vi "Set Positions.vi"(8 "error in":errorcluster, 9 "Type of Neuron":T1=enum."GC", 11 "Grid in":refnum<class "Grid.lvclass">) -> (0 "error out":errorcluster, 3 "Grid out":refnum<class "Grid.lvclass">)   [LabVIEW 2016, in "Grid.lvclass"]
doc: "This Vi perform the random allocation of #(No Nodes) inside the 3D grid of dimensions (Size(um)), accodring to the boundaries given by the Layer. Granular layer is confined to 80% in the Z dimension. Purkinje/Molecular layer is confined to 20% of the Z dimension."
uses:
  Grid.lvclass
  Controls/Type of Neuron.ctl
  Grid.lvclass/Grid.ctl
  Controls/SM Allocate Neurons.ctl
  Neuron/Neuron.lvclass/Neuron.ctl
  Neuron/Neuron.lvclass
panel:
  out "Iteration No":i32
  out "Neurons Allocated":i32
  out "Avai Ids":i32
  out "Ids Neighboor":i32[](array[numeric])
  out "Riffled {Ids}":i32[](array[numeric])
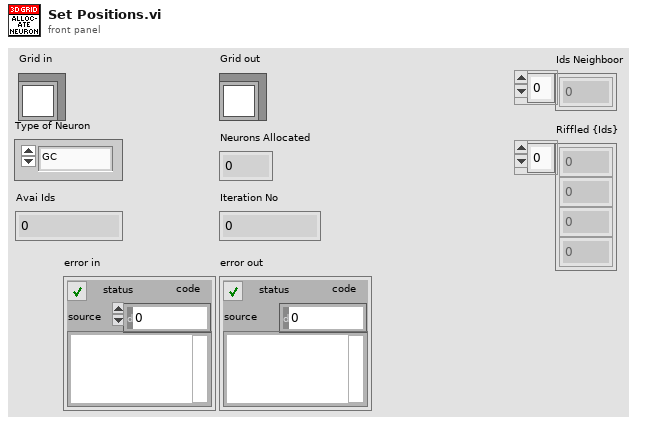
[diagram p1: front panel]
types:
  T1 = typedef "Type of Neuron.ctl" = enum16{"MF", "BA", "GO", "GC", "PC", "LU", "Glia (Dummy)"}
  T2 = typedef "SM Allocate Neurons.ctl" = enum16{"Initialize", "Generate ID", "Check Perifery", "Ocuppy it", "Stop"}
  T3 = typedef "Neuron Info.ctl" = cluster{"N":i32, "Radius":dbl, "Type":T1, "Color":u32}[]
  T4 = cluster{"N":i32, "Radius":dbl, "Type":T1, "Color":u32}
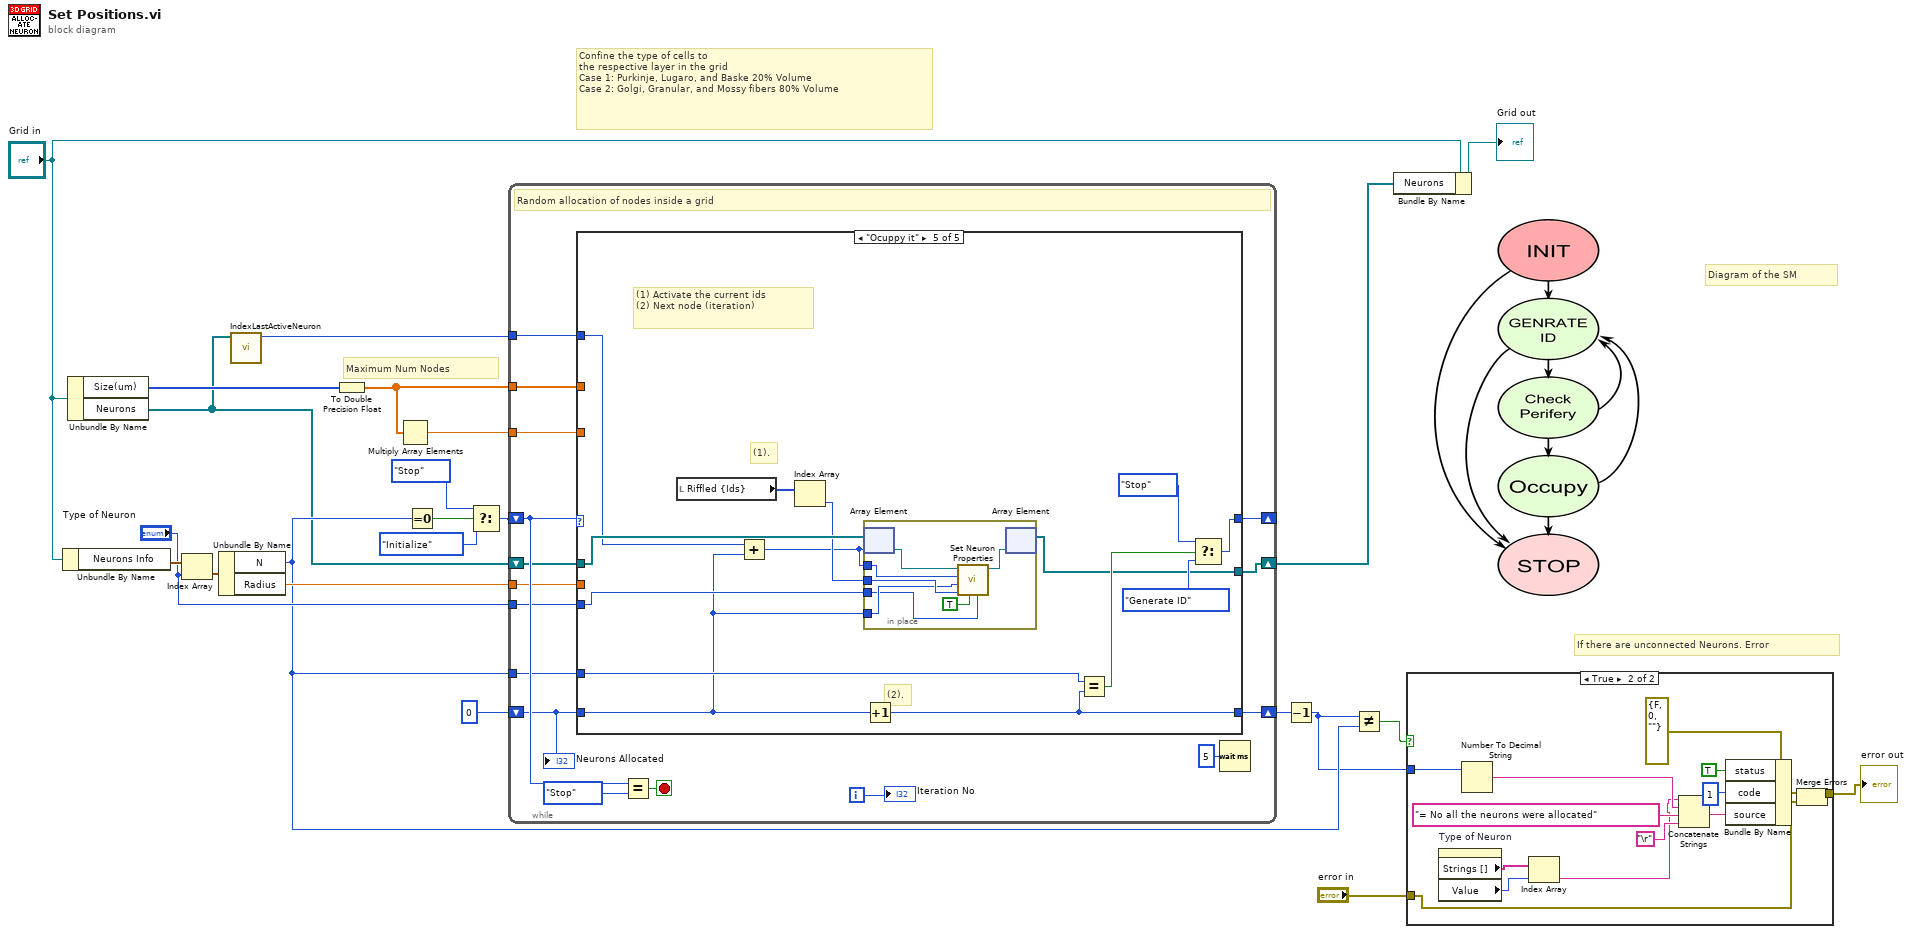
[diagram p0: block diagram]
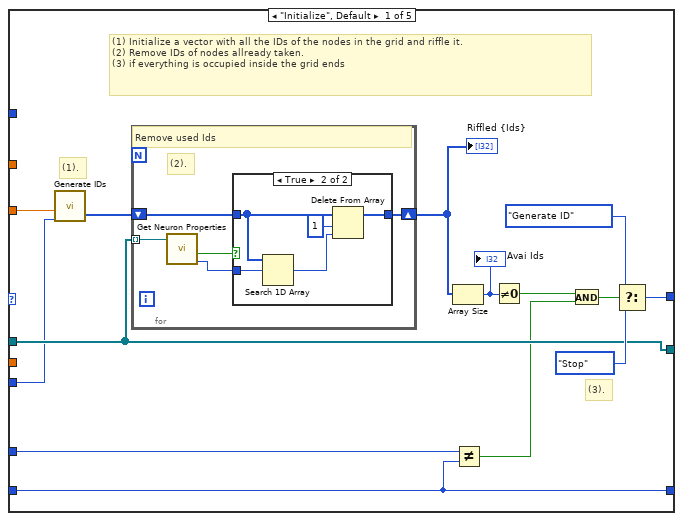
[diagram p3: hidden frame]
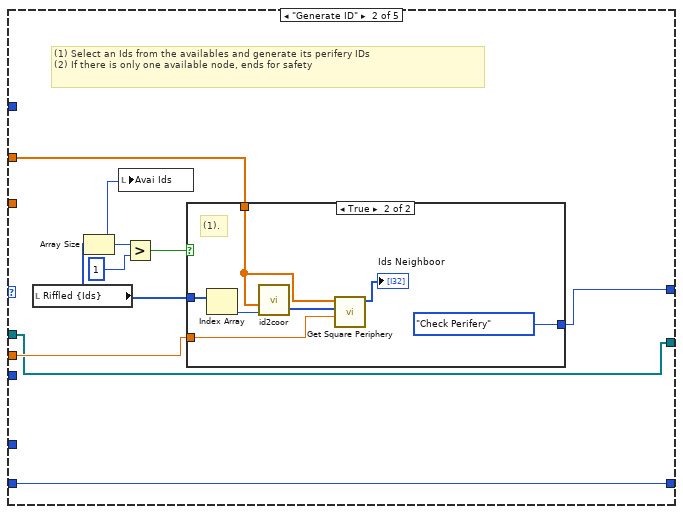
[diagram p5: hidden frame]
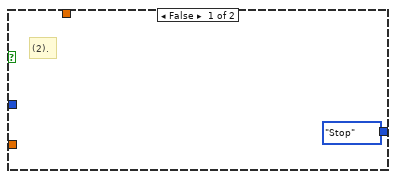
[diagram p6: hidden frame]
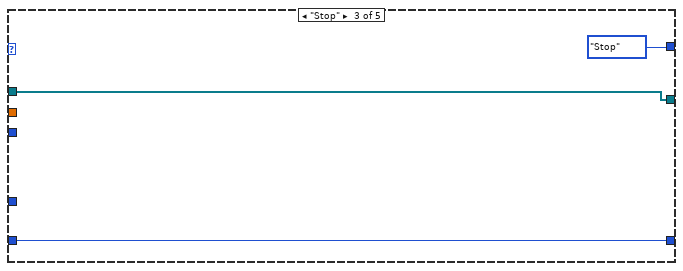
[diagram p7: hidden frame]
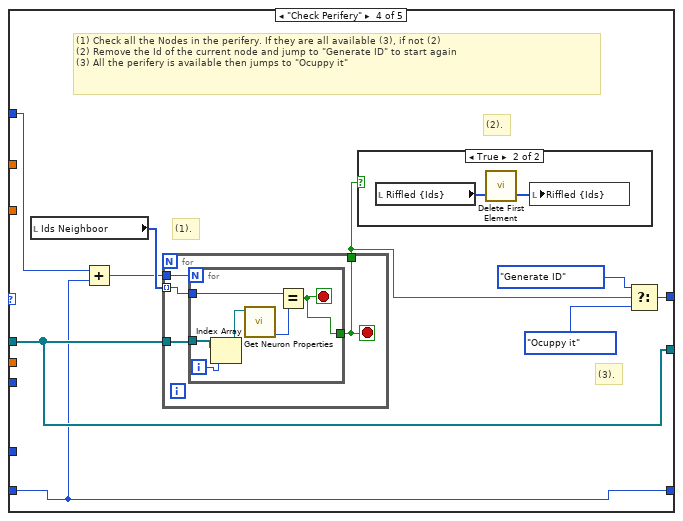
[diagram p8: hidden frame]
diagram:
  # "If there are unconnected Neurons. Error"
  # "Diagram of the SM"
  # "Confine the type of cells to \nthe respective layer in the grid\nCase 1: Purkinje, Lugaro, and Baske 20% Volume\nCase 2: Golgi, Granular, and Mossy fibers 80% Volume"
  # "Maximum Num Nodes"
  n1 = Unbundle By Name("Grid in") -> ("Neurons Info"=w20:T3)
  n2 = Unbundle By Name("Grid in") -> ("Size(um)"=w22:u32[], "Neurons"=w5:refnum<class "Neuron.lvclass">[])
  n3 = Index Array(array=w20, index="Type of Neuron") -> (element=w19:T4)
  n4 = Unbundle By Name(w19) -> ("N"=w8:i32, "Radius"=w18:dbl)
  n5 = call "IndexLastActiveNeuron.vi"("Neurons"=w5) -> ("Last Neuron"=w3:i32)  [unwired: 10 in]
  n6 = To Double Precision Float(number=w22) -> (double precision float=w13:dbl[])
  n7 = Multiply Array Elements(1:w13) -> (0:w23:dbl)
  n8 = Equal To 0?(x=w8) -> (x = 0?=w14:bool)
  n9 = Select(t=SM_Allocate_Neurons."Stop" ("Beginning State"), s=w14, f=SM_Allocate_Neurons."Initialize" ("Next State")) -> (s? t:f=w16:T2)
  n10 = while {
    shift-right: [w36] -> _
    shift-left: w16 -> [w37]
    tunnel: w23 -> [w34]
    shift-right: [w30] -> w9
    shift-left: 0 -> [w31]
    tunnel: w18 -> [w32]
    tunnel: w13 -> [w29]
    shift-right: [w28] -> w2
    shift-left: w5 -> [w33]
    tunnel: "Type of Neuron" -> [w26]
    tunnel: w8 -> [w25]
    tunnel: w3 -> [w24]
    i -> [w27]
    stop <- w39 stop-if-true
    # "Random allocation of nodes inside a grid"
    n11 = case shown="\"Ocuppy it\"" w37 {
      tunnel: [w50 w73 SM_Allocate_Neurons."Stop" ("States") w93 w116] -> w36
      tunnel: w34 -> [w44 _ _ _ _]
      tunnel: w33 -> [w48 w67 w83 w89 w118]
      tunnel: w32 -> [_ w72 _ _ _]
      tunnel: w31 -> [w40 w66 w82 w85 w109]
      tunnel: [w40 w66 w82 w85 w111] -> w30
      tunnel: w29 -> [_ w68 _ _ _]
      tunnel: [w48 w67 w83 w89 w107] -> w28
      tunnel: w26 -> [w45 _ _ _ w114]
      tunnel: w25 -> [w41 _ _ _ w112]
      tunnel: w24 -> [_ _ _ w87 w108]
      frame "Initialize", Default {
        # "(3)."
        # "(1)."
        # "(1) Initialize a vector with all the IDs of the nodes in the grid and riffle it.\n(2) Remove IDs of nodes allready taken.\n(3) if everything is occupied inside the grid ends"
        n12 = call "Generate IDs.vi"("Type of Neuron"=w45, "Size"=w44) -> ("Possible IDs"=w43:i32[])  [unwired: 5 in]
        n13 = for {
          tunnel: w48 -> [w58] mode=indexing
          shift-right: [w55] -> w53
          shift-left: w43 -> [w57]
          # "(2)."
          # "Remove used Ids"
          n14 = call "Get Neuron Properties.vi"("Neuron in"=w58) -> ("Position Key"=w56:i32, "Active"=w54:bool)  [unwired: 5 in, 4 out]
          n15 = case shown="True" w54 {
            tunnel: w57 -> [w59 w62]
            tunnel: w56 -> [_ w64]
            tunnel: [w59 w60] -> w55
            frame False {
            }
            frame True {
              n16 = Search 1D Array(1D array=w62, element=w64) -> (index of element=w63:i32)  [unwired: 1 in]
              n17 = Delete From Array(array=w62, length=1, index=w63) -> (array with subset deleted=w60:i32[])  [unwired: 1 out]
            }
          }
        }
        "Riffled {Ids}" <- w53
        n18 = Array Size(array=w53) -> (size(s)=w52:i32)
        "Avai Ids" <- w52
        n19 = Not Equal?(x=w41, y=w40) -> (x != y?=w42:bool)
        n20 = Not Equal To 0?(x=w52) -> (x != 0?=w47:bool)
        n21 = And(x=w47, y=w42) -> (x .and. y?=w46:bool)
        n22 = Select(t=SM_Allocate_Neurons."Generate ID" ("Next State"), s=w46, f=SM_Allocate_Neurons."Stop" ("Next State")) -> (s? t:f=w50:T2)
      }
      frame "Generate ID" {
        # "(1) Select an Ids from the availables and generate its perifery IDs\n(2) If there is only one available node, ends for safety"
        n23 = local read "Riffled {Ids}"() -> (w71:i32[])
        n24 = Array Size(array=w71) -> (size(s)=w65:i32)
        n25 = local write "Avai Ids"(w65) -> ()
        n26 = Greater?(x=w65, y=1) -> (0:w69:bool)
        n27 = case shown="True" w69 {
          tunnel: [SM_Allocate_Neurons."Stop" ("States") SM_Allocate_Neurons."Check Perifery" ("Next State")] -> w73
          tunnel: w71 -> [_ w80]
          tunnel: w72 -> [_ w79]
          tunnel: w68 -> [_ w77]
          frame False {
            # "(2)."
          }
          frame True {
            # "(1)."
            n28 = Index Array(array=w80) -> (element=w76:i32)  [unwired: 1 in]
            n29 = call "id2coor.vi"("Id"=w76, "Size (x,y,z)"=w77) -> ("Position (x,y,z)"=w75:i32[])  [unwired: 3 in]
            n30 = call "Get Square Periphery.vi"("Radius"=w79, "Neuron Position"=w75, "Grid Size"=w77) -> ("Square Periphery"=→"Ids Neighboor":i32[])  [unwired: 8 in]
          }
        }
      }
      frame "Stop" {
      }
      frame "Check Perifery" {
        # "(3)."
        # "(1)."
        # "(2)."
        # "(1) Check all the Nodes in the perifery. If they are all available (3), if not (2)\n(2) Remove the Id of the current node and jump to \"Generate ID\" to start again\n(3) All the perifery is available then jumps to \"Ocuppy it\""
        n31 = local read "Ids Neighboor"() -> (w90:i32[])
        n32 = Add(x=w87, y=w85) -> (x+y=w86:i32)
        n33 = for {
          tunnel: w90 -> [w95] mode=indexing
          tunnel: w89 -> [w97]
          tunnel: [w96] -> w88
          tunnel: w86 -> [w94]
          stop <- w96 stop-if-true
          n34 = for {
            N: w94 -> [_]
            tunnel: w97 -> [w100]
            tunnel: [w101] -> w96
            tunnel: w95 -> [w103]
            i -> [w99]
            stop <- w101 stop-if-true
            n35 = Index Array(array=w100, index=w99) -> (element=w98:refnum<class "Neuron.lvclass">)
            n36 = call "Get Neuron Properties.vi"("Neuron in"=w98) -> ("Position Key"=w102:i32)  [unwired: 5 in, 5 out]
            n37 = Equal?(x=w103, y=w102) -> (x = y?=w101:bool)
          }
        }
        n38 = case shown="True" w88 {
          frame False {
          }
          frame True {
            n39 = local read "Riffled {Ids}"() -> (w105:i32[])
            n40 = call "Delete First Element.vi"("Input Array"=w105) -> ("Updated Array"=w104:i32[])  [unwired: 2 in]
            n41 = local write "Riffled {Ids}"(w104) -> ()
          }
        }
        n42 = Select(t=SM_Allocate_Neurons."Generate ID" ("States"), s=w88, f=SM_Allocate_Neurons."Ocuppy it" ("States")) -> (s? t:f=w93:T2)
      }
      frame "Ocuppy it" {
        # "(2)."
        # "(1)."
        # "(1) Activate the current ids\n(2) Next node (iteration)"
        n43 = local read "Riffled {Ids}"() -> (w119:i32[])
        n44 = Add(x=w108, y=w109) -> (x+y=w106:i32)
        n45 = Index Array(array=w119) -> (element=w113:i32)  [unwired: 1 in]
        n46 = in-place {
          in-place-border: w114 -> [w120]
          in-place-border: w109 -> [w121]
          in-place-border: w113 -> [w122]
          in-place-border: w106 -> [w123]
          n47 = in-place-array #1(w118, w106) -> (w126:refnum<class "Neuron.lvclass">)
          n48 = call "Set Neuron Properties.vi"("Group"=w120, "Active"=TRUE ("Occupied"), "Position Key"=w122, "InGROUP ID"=w121, "ID"=w123, "Neuron in"=w126) -> ("Neuron out"=w125:refnum<class "Neuron.lvclass">)  [unwired: 5 in]
          n49 = in-place-array #1(w125) -> (w107:refnum<class "Neuron.lvclass">[])  [unwired: 1 out]
        }
        n50 = Increment(x=w109) -> (x+1=w111:i32)
        n51 = Equal?(x=w112, y=w111) -> (x = y?=w110:bool)
        n52 = Select(t=SM_Allocate_Neurons."Stop" ("States"), s=w110, f=SM_Allocate_Neurons."Generate ID" ("States")) -> (s? t:f=w116:T2)
      }
    }
    n53 = Equal?(x=w37, y=SM_Allocate_Neurons."Stop" ("States")) -> (x = y?=w39:bool)
    n54 = Wait (ms)(milliseconds to wait=u32 5) -> ()  [unwired: 1 out]
    "Neurons Allocated" <- w31
    "Iteration No" <- w27
  }
  n55 = Decrement(x=w9) -> (x-1=w4:i32)
  n56 = Not Equal?(x=w4, y=w8) -> (x != y?=w7:bool)
  n57 = Bundle By Name(cluster="Grid in", "Neurons"=w2) -> (→"Grid out":refnum<class "Grid.lvclass">)
  n58 = case shown="True" w7 {
    tunnel: [w127 w130] -> w11
    tunnel: w4 -> [_ w133]
    tunnel: "error in" -> [w127 w129]
    frame False {
    }
    frame True {
      n59 = property on="Type of Neuron" class="Enum (strict)"() -> ("Strings []"=w137:string[], "Value"=w136:T1)  [unwired: 2 in, 2 out]
      n60 = Number To Decimal String(number=w133) -> (decimal integer string=w132:string)  [unwired: 1 in]
      n61 = Index Array(array=w137, index=w136) -> (element=w128:string)
      n62 = Concatenate Strings(w128, w132, "= No all the neurons were allocated" ("source"), "\r") -> (w135:string)
      n63 = Bundle By Name(cluster=errorcluster {"status"=FALSE, "code"=0, "source"=""} ("error constant"), "status"=TRUE, "code"=1, "source"=w135) -> (w138:errorcluster)
      n64 = Merge Errors(w138, w129) -> (w130:errorcluster)
    }
  }
  "error out" <- w11
